vi "test -- monitor.vi"() -> ()   [LabVIEW 2012]
uses:
  cursor winow.ctl
  peak monitor ctl.ctl
  interpolation state - real.ctl
  peak -- parameters -- complex fit.ctl
  wavepacket.ctl
  filter method control.ctl
  parameters -- scan monitor control.ctl
  lorentzian.ctl
  circle corners.ctl
  cursor window action.ctl
  ctl -- name dispatcher -- action.ctl
  monitor action.ctl
  plot refs -- filter related.ctl
  next chunk - read-write freq PID file - atomic actions .vi
  ctl -- name dispatcher.vi
  Q -- check range -- i -- real.vi
  Q -- check range -- i -- real - window.vi
  Q -- check range -- i -- integer.vi
  aggregator - iii - real - atomic.vi
  switch - C.vi
  file -- 9w path.vi
  array -- find index - real.vi
  array -- interpolate -- i.vi
  Q - not nan -- real.vi
  Q - not nan -- integer.vi
  linear interpolation - real.vi
  <vilib>/Utility/libraryn.llb/Check if File or Folder Exists.vi
  file -- read list of lines.vi
  parse -- find first line.vi
  parse -- get list of matches -- numbers.vi
  Split file name.vi
  <vilib>/Utility/file.llb/Read From Spreadsheet File.vi
  <vilib>/Utility/file.llb/Read From Spreadsheet File (string).vi
  Q regex box.vi
panel:
  out "INDEX":i32
  out "Plot: phase around center":cluster{dbl[], dbl[]}[](graph)
  out "Plot: complex plane":cluster{dbl[], dbl[]}[](graph)=[{array[1409 elements], array[1409 elements]}, {[9.08730610892388e-05, 9.046915287876308e-05, 8.926379812109817e-05, 8.727600598081652e-05, 8.45371251274198e-05, 8.10903493480942e-05, 7.699003635588375e-05, 7.230085053608383e-05, 6.709674315025655e-05, 6.145978608065945e-05, 5.547887750763501e-05, 4.924833993220141e-05, 4.2866432653866014e-05, 3.6433802162774764e-05, 3.0051894884439355e-05, 2.3821357309005772e-05, 1.7840448735981335e-05, 1.2203491666384223e-05, 6.999384280556945e-06, 2.3101984607570275e-06, -1.7901145314534213e-06, -5.236890310779021e-06, -7.97577116417574e-06, -9.963563304457393e-06, -1.1168918062122294e-05, -1.1572826272598015e-05, -1.1168918062122294e-05, -9.963563304457393e-06, -7.975771164175727e-06, -5.236890310779014e-06, -1.7901145314534145e-06, 2.3101984607570343e-06, 6.999384280556959e-06, 1.220349166638425e-05, 1.7840448735981362e-05, 2.3821357309005772e-05, 3.0051894884439365e-05, 3.643380216277478e-05, 4.2866432653866034e-05, 4.924833993220145e-05, 5.5478877507634996e-05, 6.145978608065945e-05, 6.709674315025655e-05, 7.230085053608386e-05, 7.699003635588376e-05, 8.109034934809423e-05, 8.45371251274198e-05, 8.727600598081652e-05, 8.926379812109818e-05, 9.046915287876308e-05], [0.0012022998349268351, 0.001208719772091047, 0.0012150384630110944, 0.0012211562581565657, 0.0012269766762434229, 0.001232407925801487, 0.0012373643527807561, 0.0012417677913669411, 0.0012455487967030516, 0.0012486477400762733, 0.0012510157492983923, 0.001252615479449395, 0.0012534217018291677, 0.0012534217018291677, 0.001252615479449395, 0.0012510157492983923, 0.0012486477400762733, 0.0012455487967030516, 0.0012417677913669411, 0.0012373643527807561, 0.001232407925801487, 0.0012269766762434229, 0.0012211562581565657, 0.0012150384630110944, 0.001208719772091047, 0.0012022998349268351, 0.0011958798977626233, 0.0011895612068425758, 0.0011834434116971045, 0.0011776229936102474, 0.0011721917440521833, 0.0011672353170729141, 0.0011628318784867291, 0.0011590508731506187, 0.0011559519297773967, 0.001153583920555278, 0.0011519841904042752, 0.0011511779680245025, 0.0011511779680245025, 0.0011519841904042752, 0.001153583920555278, 0.001155951929777397, 0.0011590508731506187, 0.0011628318784867291, 0.0011672353170729143, 0.0011721917440521833, 0.0011776229936102474, 0.0011834434116971045, 0.0011895612068425758, 0.0011958798977626233]}, {[-7.052082546737579e-06, -2.3818625512317815e-06, 2.288357444274016e-06, 6.958577439779813e-06, 1.1628797435285612e-05, 1.629901743079141e-05, 2.0969237426297205e-05, 2.5639457421803007e-05, 3.0309677417308802e-05, 3.49798974128146e-05, 3.96501174083204e-05, 4.4320337403826194e-05, 4.899055739933199e-05, 5.366077739483779e-05, 5.833099739034359e-05, 6.300121738584938e-05, 6.767143738135518e-05, 7.234165737686099e-05, 7.701187737236677e-05, 8.168209736787258e-05], [0.0011812595288763917, 0.001183363559481436, 0.0011854675900864805, 0.0011875716206915248, 0.001189675651296569, 0.0011917796819016133, 0.0011938837125066578, 0.001195987743111702, 0.0011980917737167464, 0.0012001958043217908, 0.0012022998349268351, 0.0012044038655318794, 0.0012065078961369239, 0.0012086119267419682, 0.0012107159573470124, 0.001212819987952057, 0.0012149240185571012, 0.0012170280491621455, 0.0012191320797671898, 0.0012212361103722342]}, {[1.8609811357877078e-05, 2.071384196292141e-05, 2.281787256796574e-05, 2.492190317301007e-05, 2.70259337780544e-05, 2.9129964383098733e-05, 3.123399498814306e-05, 3.333802559318739e-05, 3.544205619823173e-05, 3.7546086803276057e-05, 3.9650117408320386e-05, 4.1754148013364715e-05, 4.3858178618409044e-05, 4.596220922345337e-05, 4.806623982849771e-05, 5.0170270433542045e-05, 5.2274301038586374e-05, 5.43783316436307e-05, 5.648236224867503e-05, 5.858639285371936e-05], [0.001249002034881893, 0.0012443318148863873, 0.0012396615948908815, 0.0012349913748953758, 0.00123032115489987, 0.001225650934904364, 0.0012209807149088582, 0.0012163104949133524, 0.0012116402749178467, 0.001206970054922341, 0.0012022998349268351, 0.0011976296149313293, 0.0011929593949358236, 0.0011882891749403178, 0.001183618954944812, 0.0011789487349493062, 0.0011742785149538003, 0.0011696082949582945, 0.0011649380749627887, 0.001160267854967283]}, {[0.13436101894698638, 0.1337313084986823, 0.13301804511574125, 0.13222167456455988, 0.13134269455080966, 0.13038165440838714, 0.1293391547560982, 0.12821584712229062, 0.1270124335376703, 0.12572966609655484, 0.12436834648683907, 0.12292932548896617, 0.12141350244421763, 0.1198218246926543, 0.11815528698105954, 0.11641493084125495, 0.11460184393917687, 0.11271715939512057, 0.11076205507557696, 0.10873775285710435], [0.024714237187312277, 0.028064574526002018, 0.03139812381741462, 0.03471280170175468, 0.03800653661324189, 0.041277270074772276, 0.04452295798439935, 0.04774157189283131, 0.05093110027114577, 0.05408954976792992, 0.057214946455060256, 0.06030533706134337, 0.06335879019324687, 0.06637339754195752, 0.06934727507601211, 0.0722785642187557, 0.07516543300989166, 0.07800607725039721, 0.08079872163008894, 0.08354162083713412]}, {[0.1540614863753245, 0.15333941839460247, 0.1525215430488301, 0.15160837148347542, 0.15060047440104185, 0.1494984817043974, 0.14830308210310603, 0.14701502268300667, 0.1456351084393087, 0.14416420177349631, 0.14260322195435557, 0.1409531445434613, 0.139215000785483, 0.13738987696369037, 0.1354789137210617, 0.13348330534741912, 0.13140429903303624, 0.129243194089185, 0.12700134113610834, 0.12468014125892643], [0.028162654665662142, 0.032004374814026376, 0.035826844668179494, 0.03962767530888943, 0.043404491340728095, 0.04715493237661627, 0.05087665451298865, 0.0545673317946573, 0.05822465766845788, 0.06184634642477037, 0.06543013462601316, 0.06897378252121779, 0.07247507544580048, 0.07593182520565536, 0.07934187144470461, 0.0827030829950506, 0.0860133592088865, 0.08927063127133286, 0.09247286349337938, 0.09561805458412452]}, {array[1409 elements], array[1409 elements]}]
  out "Plot: fragment":cluster{dbl[], dbl[]}[](graph)
  out "Plot: phase":cluster{"omega out":dbl[], dbl[]}(graph)
  out "Plot: win omega":T1(graph)
  out "Plot: dz/domega":cluster{"omega out":dbl[], dbl[]}(graph)
  in  "Plot: complex plane - filter":cluster{dbl[], dbl[]}[](graph)=[{array[1409 elements], array[1409 elements]}, {array[1409 elements], array[1409 elements]}, {[0.0002765648516185131, 0.00027612590250336593, 0.00027481078748954515, 0.00027262469673519136, 0.0002695762577417822, 0.00026567750130532524, 0.0002609438140363029, 0.00025539387763575, 0.00024904959516711475, 0.0002419360046148738, 0.00023408118007104664, 0.00022551612093957957, 0.00021627462959586136, 0.00020639317798418975, 0.00019591076367967021, 0.0001848687559826032, 0.0001733107326527555, 0.0001612823079278514, 0.0001488309525050157, 0.00013600580619561897, 0.0001228574839928925, 0.00010943787631767335, 9.579994423062008e-05, 8.199751041910182e-05, 6.808504678364034e-05, 5.411745946220482e-05, 4.014987214076934e-05, 2.623740850530786e-05, 1.2434974693789557e-05, -1.2029573932636662e-06, -1.4622565068482806e-05, -2.7770887271209277e-05, -4.059603358060599e-05, -5.304738900344177e-05, -6.507581372834585e-05, -7.66338370581935e-05, -8.767584475526055e-05, -9.815825905978006e-05, -0.00010803971067145167, -0.00011728120201516991, -0.0001258462611466369, -0.00013370108569046412, -0.00014081467624270502, -0.00014715895871134034, -0.00015270889511189323, -0.00015744258238091556, -0.00016134133881737245, -0.00016438977781078169, -0.00016657586856513542, -0.00016789098357895626, -0.00016832993269410342, -0.00016789098357895626, -0.00016657586856513542, -0.00016438977781078163, -0.00016134133881737245, -0.00015744258238091556, -0.00015270889511189318, -0.00014715895871134029, -0.00014081467624270502, -0.00013370108569046412, -0.00012584626114663685, -0.00011728120201516986, -0.00010803971067145165, -9.815825905978003e-05, -8.76758447552605e-05, -7.663383705819352e-05, -6.507581372834573e-05, -5.304738900344173e-05, -4.059603358060587e-05, -2.7770887271209236e-05, -1.4622565068482806e-05, -1.2029573932635713e-06, 1.2434974693789597e-05, 2.6237408505308004e-05, 4.0149872140769385e-05, 5.411745946220481e-05, 6.808504678364043e-05, 8.199751041910181e-05, 9.579994423062021e-05, 0.00010943787631767339, 0.00012285748399289246, 0.00013600580619561902, 0.00014883095250501567, 0.00016128230792785152, 0.00017331073265275553, 0.00018486875598260332, 0.00019591076367967032, 0.00020639317798418975, 0.00021627462959586142, 0.00022551612093957963, 0.0002340811800710467, 0.00024193600461487385, 0.00024904959516711475, 0.00025539387763575, 0.00026094381403630296, 0.0002656775013053253, 0.0002695762577417822, 0.00027262469673519136, 0.00027481078748954515, 0.00027612590250336593], [0.0012315876337959679, 0.0012455552211174034, 0.0012594676847528649, 0.001273270118564383, 0.0012869080506514364, 0.0013003276583266556, 0.001313475980529382, 0.0013263011268387786, 0.0013387524822616145, 0.0013507809069865187, 0.0013623389303163663, 0.0013733809380134332, 0.0013838633523179527, 0.0013937448039296244, 0.0014029862952733426, 0.0014115513544048096, 0.001419406178948637, 0.0014265197695008777, 0.0014328640519695132, 0.001438413988370066, 0.0014431476756390882, 0.0014470464320755453, 0.0014500948710689545, 0.001452280961823308, 0.001453596076837129, 0.0014540350259522761, 0.001453596076837129, 0.001452280961823308, 0.0014500948710689545, 0.0014470464320755453, 0.0014431476756390882, 0.0014384139883700658, 0.001432864051969513, 0.0014265197695008777, 0.001419406178948637, 0.0014115513544048096, 0.0014029862952733426, 0.0013937448039296244, 0.0013838633523179527, 0.0013733809380134332, 0.0013623389303163663, 0.0013507809069865187, 0.0013387524822616145, 0.0013263011268387786, 0.001313475980529382, 0.0013003276583266553, 0.0012869080506514364, 0.001273270118564383, 0.0012594676847528649, 0.0012455552211174034, 0.0012315876337959679, 0.0012176200464745323, 0.0012037075828390709, 0.0011899051490275527, 0.0011762672169404994, 0.0011628476092652802, 0.0011496992870625538, 0.0011368741407531571, 0.0011244227853303213, 0.0011123943606054171, 0.0011008363372755695, 0.0010897943295785023, 0.001079311915273983, 0.0010694304636623114, 0.0010601889723185931, 0.0010516239131871262, 0.0010437690886432988, 0.001036655498091058, 0.0010303112156224226, 0.0010247612792218697, 0.0010200275919528476, 0.0010161288355163905, 0.0010130803965229813, 0.0010108943057686277, 0.0010095791907548067, 0.0010091402416396596, 0.0010095791907548067, 0.0010108943057686277, 0.0010130803965229813, 0.0010161288355163905, 0.0010200275919528474, 0.00102476127922187, 0.0010303112156224226, 0.001036655498091058, 0.0010437690886432988, 0.0010516239131871262, 0.0010601889723185931, 0.0010694304636623114, 0.001079311915273983, 0.0010897943295785026, 0.0011008363372755697, 0.0011123943606054173, 0.0011244227853303213, 0.0011368741407531571, 0.0011496992870625538, 0.0011628476092652804, 0.0011762672169404994, 0.0011899051490275527, 0.001203707582839071, 0.0012176200464745323]}, {[7.767566465762977e-06, 5.411745946220485e-05, 3.7664844438504546e-08], [0.0012492522813972156, 0.0012315876337959679, 0.001210549879329941]}, {[5.0435051746976916e-05, 4.7025439630032016e-05, 4.361582751308712e-05, 4.020621539614222e-05, 3.679660327919732e-05, 3.338699116225242e-05, 2.9977379045307526e-05, 2.6567766928362625e-05, 2.3158154811417728e-05, 1.974854269447283e-05, 1.633893057752793e-05, 1.292931846058303e-05, 9.519706343638135e-06, 6.110094226693235e-06, 2.700482109748334e-06, -7.091300071965597e-07, -4.11874212414146e-06, -7.528354241086361e-06, -1.0937966358031255e-05, -1.4347578474976162e-05], [0.0012639912844977265, 0.0012623680590217138, 0.0012607448335457008, 0.0012591216080696881, 0.0012574983825936752, 0.0012558751571176625, 0.0012542519316416495, 0.0012526287061656368, 0.0012510054806896239, 0.0012493822552136111, 0.0012477590297375984, 0.0012461358042615855, 0.0012445125787855728, 0.0012428893533095598, 0.0012412661278335471, 0.0012396429023575342, 0.0012380196768815215, 0.0012363964514055085, 0.0012347732259294958, 0.0012331500004534829]}, {[5.4117459462204845e-05, 5.7876709165950375e-05, 6.163595886969591e-05, 6.539520857344144e-05, 6.915445827718697e-05, 7.29137079809325e-05, 7.667295768467805e-05, 8.043220738842356e-05, 8.419145709216911e-05, 8.795070679591464e-05, 9.170995649966017e-05, 9.54692062034057e-05, 9.922845590715123e-05, 0.00010298770561089677, 0.00010674695531464229, 0.00011050620501838783, 0.00011426545472213336, 0.0001180247044258789, 0.00012178395412962444, 0.00012554320383336996], [0.0012315876337959679, 0.0012315876337959679, 0.0012315876337959679, 0.0012315876337959679, 0.0012315876337959679, 0.0012315876337959679, 0.0012315876337959679, 0.0012315876337959679, 0.0012315876337959679, 0.0012315876337959679, 0.0012315876337959679, 0.0012315876337959679, 0.0012315876337959679, 0.0012315876337959679, 0.0012315876337959679, 0.0012315876337959679, 0.0012315876337959679, 0.0012315876337959679, 0.0012315876337959679, 0.0012315876337959679]}]
  in  "Plot: fragment - filter":cluster{dbl[], dbl[]}[](graph)=[{array[1409 elements], array[1409 elements]}, {array[1409 elements], array[1409 elements]}, {array[1409 elements], array[1409 elements]}, {array[1409 elements], array[1409 elements]}]
  out "cp lorentzian":T2={"Amplitude"=0.00016802289408286377, "omega(0)"=2645.9923573489314, "Gamma"=3.2802272186761425, "phase"=1.8816427499510646, "Q"=806.6491071971593, "Norm  Ampl"=nan, "z (inf)"=-9.117967725323189e-06+0.0011866325495290314i, "4corners"={"z (-pi/2)"=2.3982832010516637e-05+0.0012510679200604788i, "z(inf)"=-9.117967725323189e-06+0.0011866325495290314i, "z (pi/2)"=5.531740280612415e-05+0.0011535317497931915i, "z center"=3.965011740832039e-05+0.0012022998349268351i, "z(0)"=8.841820254196397e-05+0.0012179671203246388i, "radius"=5.122294368091845e-05}} {"z (inf)" format="%#9_9f"; "Q" format="%#9_9f"; "phase" format="%#9_9f"; "Gamma" format="%#9_9f"; "omega(0)" format="%#9_9f"}
  out "pm lorentzian":T2={"Amplitude"=0.00016802288350953082, "omega(0)"=2645.9923569629673, "Gamma"=3.280227012258232, "phase"=1.994083151681052, "Q"=806.6491578402575, "Norm  Ampl"=nan, "z (inf)"=-7.052082546737586e-06+0.0011812595288763917i, "4corners"={"z (-pi/2)"=1.860981135787708e-05+0.001249002034881893i, "z(inf)"=-7.052082546737586e-06+0.0011812595288763917i, "z (pi/2)"=6.06904234587637e-05+0.0011555976349717772i, "z center"=3.965011740832039e-05+0.0012022998349268351i, "z(0)"=8.635231736337838e-05+0.0012233401409772785i, "radius"=5.122294368091841e-05}} {"z (inf)" format="%#9_9f"; "Q" format="%#9_9f"; "phase" format="%#9_9f"; "Gamma" format="%#9_9f"; "omega(0)" format="%#9_9f"}
  in  "scan monitor control":T4={"gamma acc. - min "=0.7, "gamma acc. - max"=1.4, "peak acc. fraction"=2.0, "min peak acc. window (kHz)"=0.1, "use"=enum."fraction", "abs gamma min(kHz)"=0.01, "abs gamma max(kHz)"=10.0, "# point in linear"=7, "gamma-factor"=2.0, "interpolate"=enum."last", "init linear"=FALSE, "global"=TRUE, "max peak acc. window (kHz)"=10.0}
  in  "parameters: complex fit":T5={"main VI path"=path "E:/ProjectLocker/LANL/Libraries/control rus sweep -- library/monitor RUS scan.vi", "scale factor"=3.0, "# of grid points"=150, "parameters: wavepacket"={"R"=0.5, "wave number"=22.0, "delta k"=7.0, "radii vector"=[], "radial section"=[], "wave vector"=22.0, "wavepacket is"=TRUE}, "span"=0.33799, "interference ?"=enum."pm zcenter", "filter method"=enum."three"} {"span" min=0.0 max=0.5 step=1e-05 scale=0.0001..0.5 scale format="%#_5f"; "parameters: wavepacket"."delta k" format="%#_3f"; "parameters: wavepacket"."wave number" format="%#_3f"; "parameters: wavepacket"."R" format="%#_3f"}
  in  "plot what":enum16{"plot pm", "plot cp", "a"}(ring)
  out "peaks OK":bool
  in  "iterate #":i32=2000
  out "# points in window":dbl=1408.8856011517964
  in  "plot staff":enum16{"plot", "do not plot", "a"}(ring)=enum."do not plot"
  in  "Array":T8[](array[typedef])=[{"delta"=0.0, "gamma"=0.7984180708092088, "exp"=573.2171646782067, "found?"=TRUE, "found"=573.2171646782067, "gamma found"=0.7984180708092088, "init linear"=FALSE, "interpolate"=enum."line", "gamma-factor"=2.0, "slope"=0.0, "linear interpolation state"={"requested size"=7, "Array"=[573.2171646782067, 573.2171646782067, 573.2171646782067, 573.2171646782067, 573.2171646782067, 573.2171646782067, 573.2171646782067], "actual number of elements"=7}, "update freq?"=TRUE, "update gamma?"=TRUE, "acc factor"=3.5}, {"delta"=-0.00016990006724881823, "gamma"=0.7626775564883673, "exp"=764.2078782920015, "found?"=TRUE, "found"=764.2077083919343, "gamma found"=0.7635570706743358, "init linear"=FALSE, "interpolate"=enum."line", "gamma-factor"=2.0, "slope"=7.424446545085128e-14, "linear interpolation state"={"requested size"=7, "Array"=[764.2077083919343, 764.2077083919343, 764.2077083919343, 764.2077083919343, 764.2077083919343, 764.2077083919343, 764.2077083919343], "actual number of elements"=7}, "update freq?"=TRUE, "update gamma?"=TRUE, "acc factor"=3.5}, {"delta"=0.0, "gamma"=0.9481310196462865, "exp"=1002.0694247582248, "found?"=TRUE, "found"=1002.0694247582248, "gamma found"=0.9481310196462865, "init linear"=FALSE, "interpolate"=enum."line", "gamma-factor"=2.0, "slope"=2.4138535824319235e-06, "linear interpolation state"={"requested size"=7, "Array"=[1002.0694247582248, 1002.0694022289256, 1002.0694022289256, 1002.0694022289256, 1002.0694247582248, 1002.0694247582248, 1002.0694247582248], "actual number of elements"=7}, "update freq?"=TRUE, "update gamma?"=TRUE, "acc factor"=3.5}, {"delta"=0.0, "gamma"=1.6163366783885946, "exp"=1178.9533054882218, "found?"=TRUE, "found"=1178.9533054882218, "gamma found"=1.6163366783885946, "init linear"=FALSE, "interpolate"=enum."line", "gamma-factor"=2.0, "slope"=1.4848893090170256e-13, "linear interpolation state"={"requested size"=7, "Array"=[1178.9533054882218, 1178.9533054882218, 1178.9533054882218, 1178.9533054882218, 1178.9533054882218, 1178.9533054882218, 1178.9533054882218], "actual number of elements"=7}, "update freq?"=TRUE, "update gamma?"=TRUE, "acc factor"=3.5}, {"delta"=-5.7470326964903506e-05, "gamma"=0.5065402785323723, "exp"=1304.5805431106835, "found?"=TRUE, "found"=1304.5804856403565, "gamma found"=0.5029497047898763, "init linear"=FALSE, "interpolate"=enum."line", "gamma-factor"=2.0, "slope"=-0.00011420019018260064, "linear interpolation state"={"requested size"=7, "Array"=[0.0, 0.0, 0.0, 0.0, 0.0, 1304.5805998405465, 1304.5804856403565], "actual number of elements"=2}, "update freq?"=TRUE, "update gamma?"=TRUE, "acc factor"=3.5}, {"delta"=0.0, "gamma"=0.44981224983108903, "exp"=1576.6403877708215, "found?"=TRUE, "found"=1576.6403877708215, "gamma found"=0.44981224983108903, "init linear"=FALSE, "interpolate"=enum."line", "gamma-factor"=2.0, "slope"=0.0, "linear interpolation state"={"requested size"=7, "Array"=[1576.6403877708215, 1576.6403877708215, 1576.6403877708215, 1576.6403877708215, 1576.6403877708215, 1576.6403877708215, 1576.6403877708215], "actual number of elements"=7}, "update freq?"=TRUE, "update gamma?"=TRUE, "acc factor"=3.5}, {"delta"=0.0, "gamma"=1.4980549364226101, "exp"=1600.0388900188668, "found?"=TRUE, "found"=1600.0388900188668, "gamma found"=1.4980549364226101, "init linear"=FALSE, "interpolate"=enum."line", "gamma-factor"=2.0, "slope"=2.969778618034051e-13, "linear interpolation state"={"requested size"=7, "Array"=[1600.0388900188668, 1600.0388900188668, 1600.0388900188668, 1600.0388900188668, 1600.0388900188668, 1600.0388900188668, 1600.0388900188668], "actual number of elements"=7}, "update freq?"=TRUE, "update gamma?"=TRUE, "acc factor"=3.5}, {"delta"=0.0, "gamma"=2.044217926576064, "exp"=1686.988927244952, "found?"=TRUE, "found"=1686.988927244952, "gamma found"=2.044217926576064, "init linear"=FALSE, "interpolate"=enum."line", "gamma-factor"=2.0, "slope"=-1.4848893090170256e-13, "linear interpolation state"={"requested size"=7, "Array"=[1686.988927244952, 1686.988927244952, 1686.988927244952, 1686.988927244952, 1686.988927244952, 1686.988927244952, 1686.988927244952], "actual number of elements"=7}, "update freq?"=TRUE, "update gamma?"=TRUE, "acc factor"=3.5}, {"delta"=0.0, "gamma"=0.9751532640186273, "exp"=1821.560752570059, "found?"=TRUE, "found"=1821.560752570059, "gamma found"=0.9751532640186273, "init linear"=FALSE, "interpolate"=enum."line", "gamma-factor"=2.0, "slope"=0.0, "linear interpolation state"={"requested size"=7, "Array"=[1821.560752570059, 1821.560752570059, 1821.560752570059, 1821.560752570059, 1821.560752570059, 1821.560752570059, 1821.560752570059], "actual number of elements"=7}, "update freq?"=TRUE, "update gamma?"=TRUE, "acc factor"=3.5}, {"delta"=0.0, "gamma"=0.8978096293996316, "exp"=1941.7641922241392, "found?"=TRUE, "found"=1941.7641922241392, "gamma found"=0.8978096293996316, "init linear"=FALSE, "interpolate"=enum."line", "gamma-factor"=2.0, "slope"=0.0, "linear interpolation state"={"requested size"=7, "Array"=[1941.7641922241392, 1941.7641922241392, 1941.7641922241392, 1941.7641922241392, 1941.7641922241392, 1941.7641922241392, 1941.7641922241392], "actual number of elements"=7}, "update freq?"=TRUE, "update gamma?"=TRUE, "acc factor"=3.5}, {"delta"=0.0008234488909693027, "gamma"=7.6645915516534995, "exp"=2228.416486556786, "found?"=TRUE, "found"=2228.417310005677, "gamma found"=7.700686103199007, "init linear"=FALSE, "interpolate"=enum."line", "gamma-factor"=2.0, "slope"=8.822666696149248e-05, "linear interpolation state"={"requested size"=7, "Array"=[2228.416486556786, 2228.417310005677, 2228.417310005677, 2228.417310005677, 2228.417310005677, 2228.417310005677, 2228.417310005677], "actual number of elements"=7}, "update freq?"=TRUE, "update gamma?"=TRUE, "acc factor"=3.5}, {"delta"=-0.00013044922297922312, "gamma"=2.03557905656649, "exp"=2288.7421723268762, "found?"=TRUE, "found"=2288.7420418776533, "gamma found"=2.024887078708222, "init linear"=FALSE, "interpolate"=enum."line", "gamma-factor"=2.0, "slope"=0.0, "linear interpolation state"={"requested size"=7, "Array"=[2288.7420418776533, 2288.7420418776533, 2288.7420418776533, 2288.7420418776533, 2288.7420418776533, 2288.7420418776533, 2288.7420418776533], "actual number of elements"=7}, "update freq?"=TRUE, "update gamma?"=TRUE, "acc factor"=3.5}, {"delta"=0.0012348836899036542, "gamma"=5.364259019853043, "exp"=2340.875532010553, "found?"=TRUE, "found"=2340.876766894243, "gamma found"=5.340243230177507, "init linear"=FALSE, "interpolate"=enum."line", "gamma-factor"=2.0, "slope"=3.813747678911884e-05, "linear interpolation state"={"requested size"=7, "Array"=[2340.876766894243, 2340.875532010553, 2340.876599859903, 2340.876766894243, 2340.875532010553, 2340.876599859903, 2340.876766894243], "actual number of elements"=7}, "update freq?"=TRUE, "update gamma?"=TRUE, "acc factor"=3.5}, {"delta"=0.0, "gamma"=1.7924026784773852, "exp"=2387.980805890703, "found?"=TRUE, "found"=2387.980805890703, "gamma found"=1.7924026784773852, "init linear"=FALSE, "interpolate"=enum."line", "gamma-factor"=2.0, "slope"=-2.969778618034051e-13, "linear interpolation state"={"requested size"=7, "Array"=[2387.980805890703, 2387.980805890703, 2387.980805890703, 2387.980805890703, 2387.980805890703, 2387.980805890703, 2387.980805890703], "actual number of elements"=7}, "update freq?"=TRUE, "update gamma?"=TRUE, "acc factor"=3.5}, {"delta"=-0.0037933986345706217, "gamma"=3.2891295717771207, "exp"=2645.996150361602, "found?"=TRUE, "found"=2645.9923569629673, "gamma found"=3.280227012258232, "init linear"=FALSE, "interpolate"=enum."line", "gamma-factor"=2.0, "slope"=-0.00028348227841684556, "linear interpolation state"={"requested size"=7, "Array"=[2645.9936798802655, 2645.9936798802655, 2645.9936798802655, 2645.9936798802655, 2645.9923569629673, 2645.9923569629673, 2645.9923569629673], "actual number of elements"=7}, "update freq?"=TRUE, "update gamma?"=TRUE, "acc factor"=3.5}]
  in  "cursor bracket: All, data window":T10={"left"=2642.7070207898246, "right "=2649.285279933379, "center"=2645.996150361602, "window"=6.5782591435542415, "cursors"=[0, 1, 2], "relative"=0, "absolute"=0, "fixed vertical offset"=0.0, "vertical offset"=0.0, "skew"=0.0, "default window frac"=0.1, "kind"=enum."symmetric", "skew.left"=0.5, "skew.right"=0.5, "Plot ref"=refnum, "wing order"=enum."back"}
  in  "file path":path=path "E:/data/Ultrasound/Experiment/ProbeTest/Probe10/YBCO_6/sweep4/August_2012/081512/298.62200K_200_3500_001_081512.bin"
  in  "temperature":dbl=298.622
  in  "Sweep folder path":path=path "E:/data/Ultrasound/Experiment/ProbeTest/Probe10/YBCO_6/sweep3"
  in  "source":enum16{"last scan file", "manual"}(ring)
  out "scan file found":bool=TRUE
  out "Plot: All":cluster{"all rows":dbl[], "all rows":dbl[]}[](graph)
  out "all:max omega":dbl=2723.224510691464
  out "all:min omega":dbl=205.0
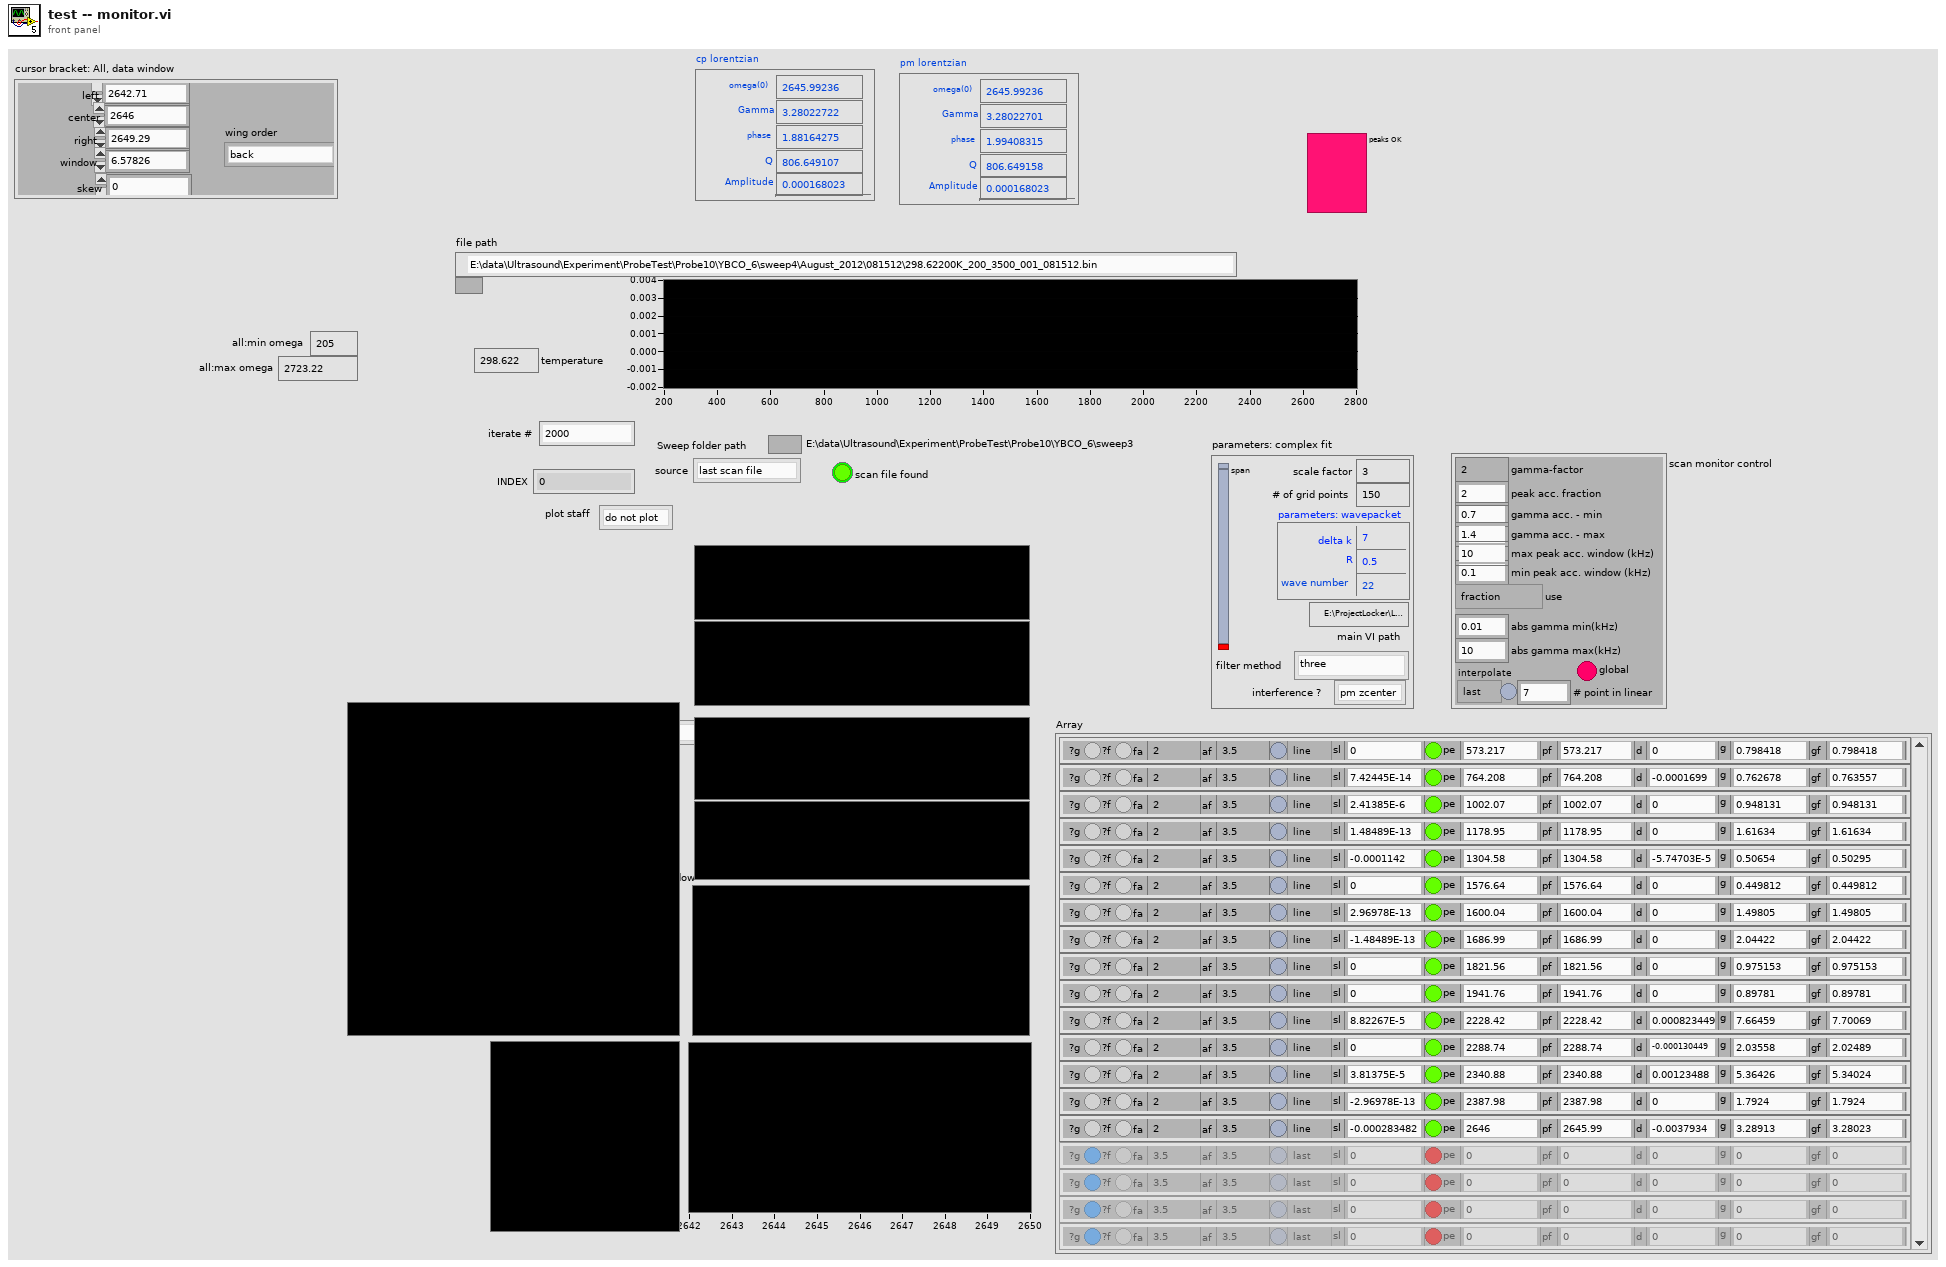
[diagram p1: front panel]
types:
  T1 = cluster{"omega out":dbl[], "win omega out":dbl[]}
  T2 = typedef "lorentzian.ctl" = cluster{"Amplitude":dbl, "omega(0)":dbl, "Gamma":dbl, "phase":dbl, "Q":dbl, "Norm  Ampl":dbl, "z (inf)":cdb, "4corners":T3}
  T3 = typedef "circle corners.ctl" = cluster{"z (-pi/2)":cdb, "z(inf)":cdb, "z (pi/2)":cdb, "z center":cdb, "z(0)":cdb, "radius":dbl}
  T4 = typedef "parameters -- scan monitor control.ctl" = cluster{"gamma acc. - min ":dbl, "gamma acc. - max":dbl, "peak acc. fraction":dbl, "min peak acc. window (kHz)":dbl, "use":enum16{"window", "fraction"}, "abs gamma min(kHz)":dbl, "abs gamma max(kHz)":dbl, "# point in linear":i32, "gamma-factor":dbl, "interpolate":enum16{"line", "last"}, "init linear":bool, "global":bool, "max peak acc. window (kHz)":dbl}
  T5 = typedef "peak -- parameters -- complex fit.ctl" = cluster{"main VI path":path, "scale factor":dbl, "# of grid points":i32, "parameters: wavepacket":T6, "span":dbl, "interference ?":enum16{"cp z center", "pm zcenter", "fancy"}, "filter method":T7}
  T6 = typedef "wavepacket.ctl" = cluster{"R":dbl, "wave number":dbl, "delta k":dbl, "radii vector":dbl[], "radial section":cdb[], "wave vector":dbl, "wavepacket is":bool}
  T7 = typedef "filter method control.ctl" = enum16{"four", "five", "one", "two", "three", "zero", "minus one", "minus two"}
  T8 = typedef "peak monitor ctl.ctl" = cluster{"delta":dbl, "gamma":dbl, "exp":dbl, "found?":bool, "found":dbl, "gamma found":dbl, "init linear":bool, "interpolate":enum16{"line", "last"}, "gamma-factor":dbl, "slope":dbl, "linear interpolation state":T9, "update freq?":bool, "update gamma?":bool, "acc factor":dbl}
  T9 = typedef "interpolation state - real.ctl" = cluster{"requested size":i32, "Array":dbl[], "actual number of elements":i32}
  T10 = typedef "cursor winow.ctl" = cluster{"left":dbl, "right ":dbl, "center":dbl, "window":dbl, "cursors":i32[], "relative":i32, "absolute":i32, "fixed vertical offset":dbl, "vertical offset":dbl, "skew":dbl, "default window frac":dbl, "kind":enum16{"symmetric", "skewed", "fancy"}, "skew.left":dbl, "skew.right":dbl, "Plot ref":refnum<vi>, "wing order":enum16{"forw", "back"}}
  T11 = typedef "plot refs -- filter related.ctl" = cluster{"Plot: complex plane - filter":refnum<vi>, "Plot: dz/domega":refnum<vi>, "Plot: fragment filter":refnum<vi>, "Plot: win omega":refnum<vi>, "Plot: phase":refnum<vi>, "Plot: phase around center":refnum<vi>, "Plot: complex plane":refnum<vi>, "Plot: fragment":refnum<vi>}
  T12 = typedef "monitor action.ctl" = enum16{"monitor", "interpolate", "global", "nothing"}
  T13 = typedef "ctl -- name dispatcher -- action.ctl" = enum16{"peak frequency", "peak frequency DUMP", "peak gamma DUMP", "peak gamma", "peak frequency TEST", "peak gamma TEST", "ultrasonic power", "time in gamma", "set temperature ", "set temperature timer", "peak default gamma", "last scan file", "peak freq gamma TEST", "peak NAMES", "errors", "P_I_D", "P", "I", "D"}
  T14 = typedef "cursor window action.ctl" = enum16{"balance", "h. offset change", "cursor moves", "change center", "change window", "init", "check", "reset", "set y to middle", "idle", "-write all Y", "-write left.X", "-write center.X", "-write right.X", "-write all X", "-change center", "-change window", "-change skew", "-read cursor 2", "-read cursor 1", "-read cursor 0", "-read all cursors", "-reset", "-read plot scale", "-set y to middle", "-Q: center.Y is visible", "-Q: window is visible", "-parse center.Y", "-right left from center", "-left move", "-right move", "-set center.Y", "-empty", "-set cursors to default", "-check", "-write center.Y", "-copy cursor 1", "-copy cursor 0", "-copy cursor 2", "move right", "move left", "shrink", "broaden", "skew up", "skew down", "-write plot scale", "zoom X", "change cen&win"}
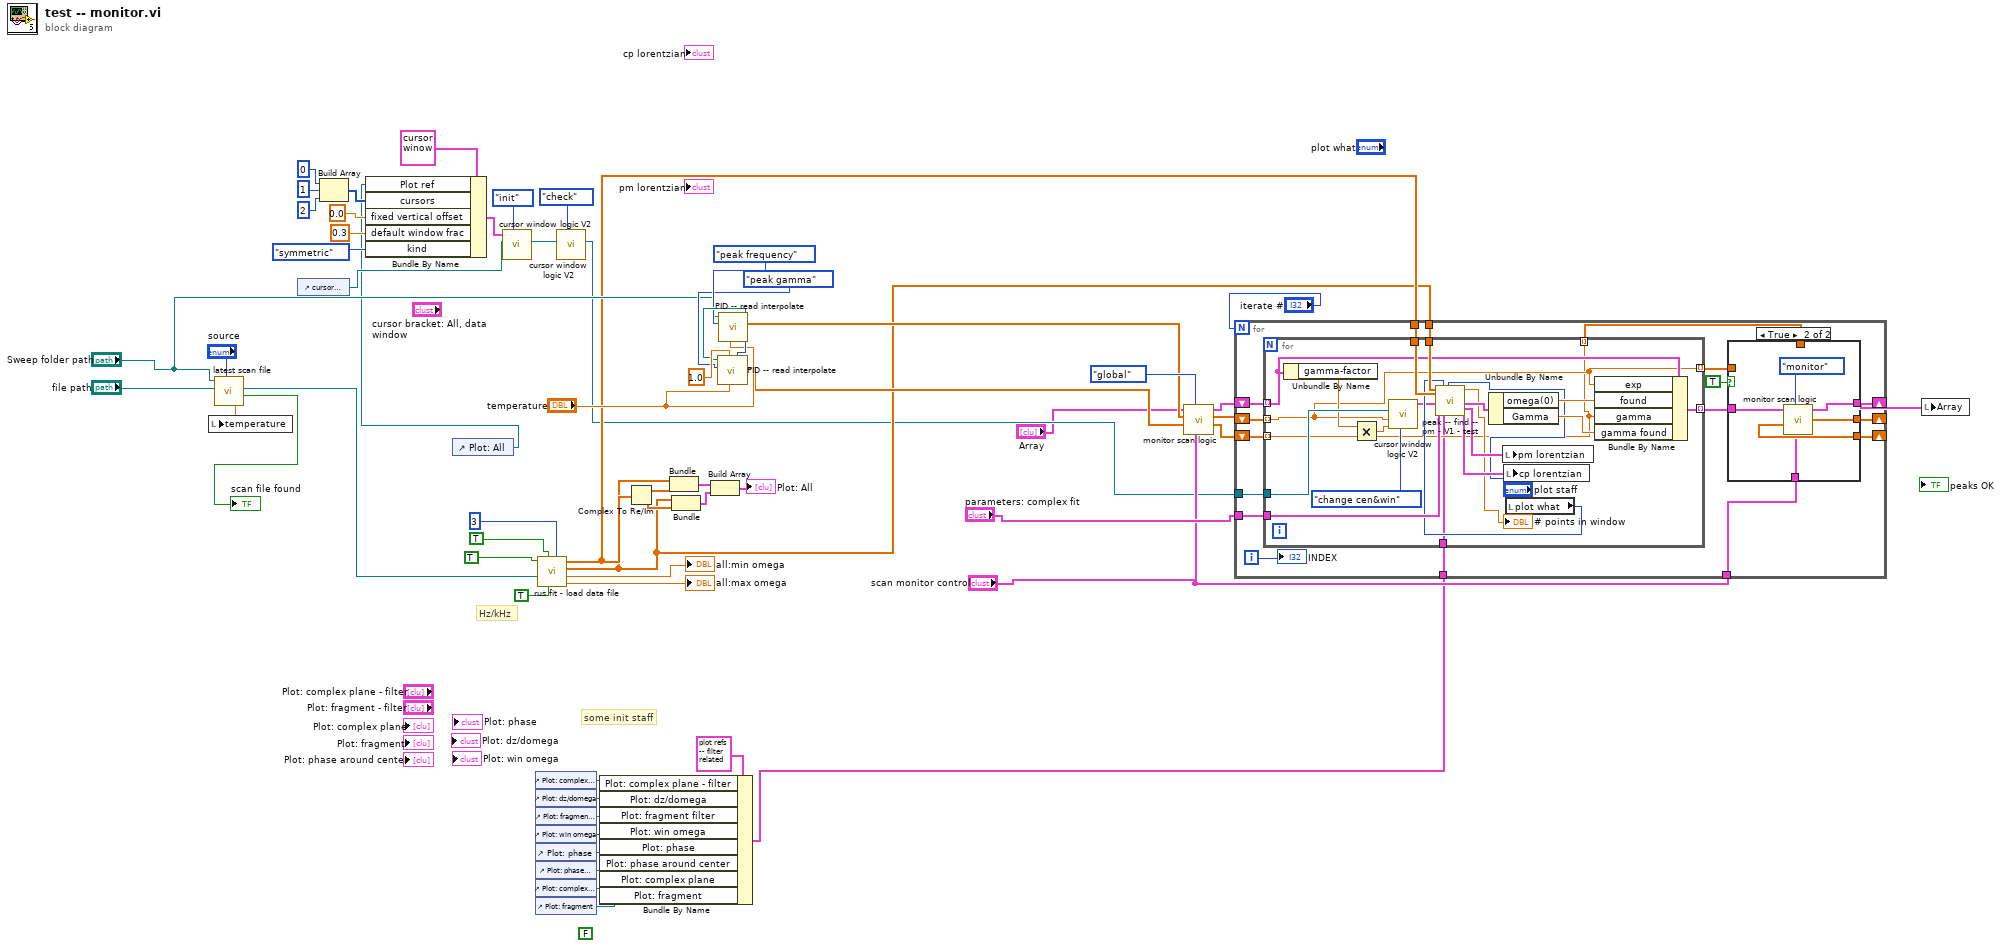
[diagram p0: block diagram]
diagram:
  (unwired) FALSE
  # "some init staff"
  # "Hz/kHz"
  n1 = call "latest scan file.vi"("source"="source", "file path in"="file path", "sweep folder"="Sweep folder path") -> ("temperature"=w60:dbl, "file or folder exists?"=→"scan file found":bool, "file path out"=w29:path)  [unwired: 6 in]
  n2 = local write "temperature"(w60) -> ()
  n3 = control-ref of="cursor bracket: All, data window"() -> (w13:refnum<vi>)
  n4 = Build Array(0, 1, 2) -> (w47:i32[])
  n5 = control-ref of="Plot: All"() -> (w12:refnum<vi>)
  n6 = Bundle By Name(cluster=T10 {"left"=3014.1710549361324, "right "=3018.2569539294045, "center"=3016.2140044327684, "window"=4.085898993271756, "cursors"=[0, 1, 2], "relative"=0, "absolute"=0, "fixed vertical offset"=0.0, "vertical offset"=0.0, "skew"=0.0, "default window frac"=0.1, "kind"=enum."skewed", "skew.left"=0.5, "skew.right"=0.5, "Plot ref"=refnum, "wing order"=enum."back"} ("cursor bracket: All, data window"), "Plot ref"=w12, "cursors"=w47, "fixed vertical offset"=0.0, "default window frac"=0.3 ("fixed vertical offset"), "kind"=enum16{"symmetric", "skewed", "fancy"}."symmetric") -> (w39:T10)
  n7 = call "cursor window logic V2.vi"("cursor window action"=cursor_window_action."init", "cursor window in"=w13, "cursor window init"=w39) -> ("cursor window out"=w37:refnum<vi>)  [unwired: 7 in, 1 out]
  n8 = control-ref of="Plot: complex plane - filter"() -> (w9:refnum<vi>)
  n9 = control-ref of="Plot: dz/domega"() -> (w8:refnum<vi>)
  n10 = control-ref of="Plot: fragment - filter"() -> (w7:refnum<vi>)
  n11 = control-ref of="Plot: win omega"() -> (w6:refnum<vi>)
  n12 = control-ref of="Plot: phase"() -> (w5:refnum<vi>)
  n13 = control-ref of="Plot: phase around center"() -> (w4:refnum<vi>)
  n14 = control-ref of="Plot: complex plane"() -> (w3:refnum<vi>)
  n15 = control-ref of="Plot: fragment"() -> (w2:refnum<vi>)
  n16 = call "rus fit - load data file.vi"("number of columns in the binary file"=3 ("# columns in bin file"), "read freq in"=TRUE, "create bin file when only dat file is present"=TRUE ("create bin file from dat"), "file path"=w29, "phase is normalized"=TRUE) -> ("all:max omega"=→"all:max omega":dbl, "all:min omega"=→"all:min omega":dbl, "omega"=w17:dbl[], "x + iy"=w18:cdb[])  [unwired: 2 in, 1 out]
  n17 = call "cursor window logic V2.vi"("cursor window action"=cursor_window_action."check", "cursor window in"=w37) -> ("cursor window out"=w16:refnum<vi>)  [unwired: 8 in, 1 out]
  n18 = Bundle By Name(cluster=T11 {"Plot: complex plane - filter"=refnum, "Plot: dz/domega"=refnum, "Plot: fragment filter"=refnum, "Plot: win omega"=refnum, "Plot: phase"=refnum, "Plot: phase around center"=refnum, "Plot: complex plane"=refnum, "Plot: fragment"=refnum} ("plots: filter related"), "Plot: complex plane - filter"=w9, "Plot: dz/domega"=w8, "Plot: fragment filter"=w7, "Plot: win omega"=w6, "Plot: phase"=w5, "Plot: phase around center"=w4, "Plot: complex plane"=w3, "Plot: fragment"=w2) -> (w1:T11)
  n19 = Complex To Re/Im(x + iy=w18) -> (x=w50:dbl[], y=w49:dbl[])
  n20 = Bundle("omega"=w17, w50) -> (w51:cluster{"omega":dbl[], dbl[]})  [unwired: 1 in]
  n21 = Bundle("omega"=w17, w49) -> (w52:cluster{"omega":dbl[], dbl[]})  [unwired: 1 in]
  n22 = Build Array(w51, w52) -> (→"Plot: All":cluster{"omega":dbl[], dbl[]}[])
  n23 = call "PID -- read interpolate.vi"("temperature"="temperature", "ctl PID file IN"=ctl_--_name_dispatcher_--_action."peak frequency" ("ctl name dispatch"), "sweep folder path"="Sweep folder path") -> ("length out"=w34:i32, "PID freq"=w22:dbl[], "sweep folder path out"=w33:path)  [unwired: 4 in, 2 out]
  n24 = call "PID -- read interpolate.vi"("length"=w34, "temperature"="temperature", "default"=1.0 ("element"), "ctl PID file IN"=ctl_--_name_dispatcher_--_action."peak gamma" ("ctl name dispatch"), "sweep folder path"=w33) -> ("PID freq"=w21:dbl[])  [unwired: 2 in, 4 out]
  n25 = call "monitor scan logic.vi"("scan monitor control"="scan monitor control", "monitor action"=monitor_action."global", "new gamma IN"=w21, "new freq IN"=w22, "Array"="Array") -> ("new gamma"=w24:dbl[], "new freq"=w23:dbl[], "Array out"=w26:T8[])  [unwired: 3 in, 1 out]
  n26 = for {
    N: "iterate #" -> [_]
    tunnel: w17 -> [w78]
    tunnel: w18 -> [w77]
    tunnel: w16 -> [w76]
    tunnel: "parameters: complex fit" -> [w71]
    tunnel: "scan monitor control" -> [w70]
    shift-right: [w68] -> _
    shift-left: w23 -> [w74]
    shift-right: [w73] -> _
    shift-left: w24 -> [w69]
    shift-right: [w72] -> w14
    shift-left: w26 -> [w67]
    tunnel: w1 -> [w62]
    i -> [w66]
    n27 = for {
      tunnel: w74 -> [w90] mode=indexing
      tunnel: w76 -> [w108]
      tunnel: w78 -> [w102]
      tunnel: w77 -> [w101]
      tunnel: [w106] -> w75 mode=indexing
      tunnel: w69 -> [w89] mode=indexing
      tunnel: w71 -> [w99]
      tunnel: w67 -> [w92] mode=indexing
      tunnel: [w90] -> w64 mode=indexing
      tunnel: [w89] -> w63 mode=indexing
      tunnel: w62 -> [w88]
      n28 = Unbundle By Name(w92) -> ("gamma-factor"=w91:dbl)
      n29 = Multiply(x=w91, y=w89) -> (x*y=w105:dbl)
      n30 = call "cursor window logic V2.vi"("cursor window action"=cursor_window_action."change cen&win", "window"=w105, "center"=w90, "cursor window in"=w108) -> ("cursor window out"=w95:T10)  [unwired: 6 in, 1 out]
      n31 = local read "plot what"() -> (w96:enum16{"plot pm", "plot cp", "a"})
      n32 = call "peak -- find -- pm - V1 - test.vi"("omega in"=w102, "z in"=w101, "cursor window"=w95, "parameters: complex fit"=w99, "plot what"=w96, "plots: filter related"=w88, "plot staff"="plot staff") -> ("# points in window"=→"# points in window":dbl, "good lorentzian"=w97:T2, "pm lorentzian"=w103:T2, "cp lorentzian"=w98:T2)  [unwired: 9 in]
      n33 = Unbundle By Name(w97) -> ("omega(0)"=w100:dbl, "Gamma"=w104:dbl)
      n34 = local write "pm lorentzian"(w103) -> ()
      n35 = local write "cp lorentzian"(w98) -> ()
      n36 = Bundle By Name(cluster=w92, "exp"=w90, "found"=w100, "gamma"=w89, "gamma found"=w104) -> (w106:T8)
    }
    n37 = case shown="True" TRUE {
      tunnel: w75 -> [w79 w87]
      tunnel: [w80 w86] -> w73
      tunnel: [w79 w85] -> w72
      tunnel: w70 -> [_ w84]
      tunnel: [w81 w83] -> w68
      tunnel: w64 -> [w81 _]
      tunnel: w63 -> [w80 _]
      frame False {
      }
      frame True {
        n38 = call "monitor scan logic.vi"("scan monitor control"=w84, "monitor action"=monitor_action."monitor", "Array"=w87) -> ("new gamma"=w86:dbl[], "new freq"=w83:dbl[], "Array out"=w85:T8[])  [unwired: 5 in, 1 out]
      }
    }
    "INDEX" <- w66
  }
  n39 = local write "Array"(w14) -> ()
